vi "Array Outer Product (1D x 1D).vi"(1 "array a":dbl[](array[numeric])=[2.0, 1.0, 3.0], 4 "array b":dbl[](array[numeric])=[1.0, 2.0, 3.0]) -> (15 "a X b":dbl[][](array[numeric])=[[2.0, 4.0, 6.0], [1.0, 2.0, 3.0], [3.0, 6.0, 9.0]])   [LabVIEW 2014]
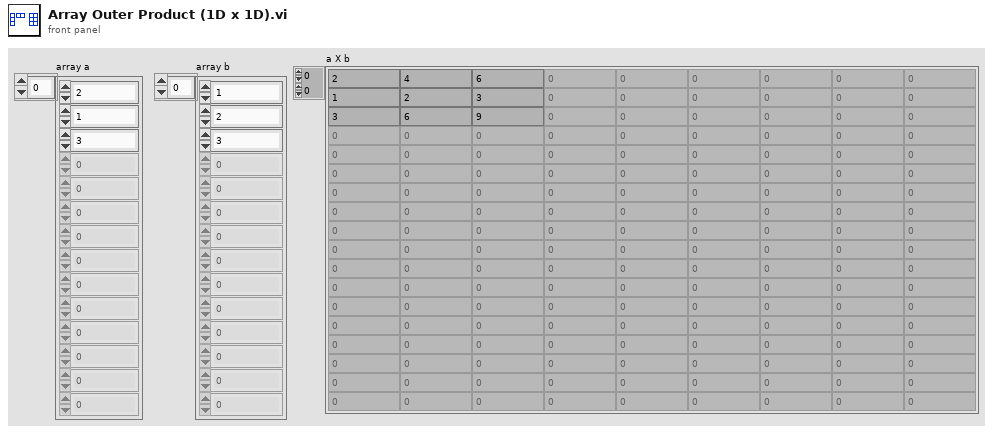
[diagram p1: front panel]
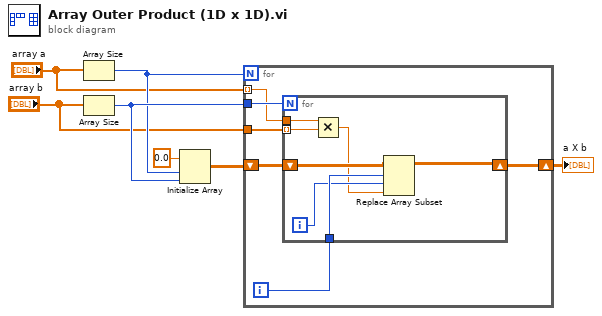
[diagram p0: block diagram]
diagram:
  n1 = Array Size(array="array a") -> (size(s)=w5:i32)
  n2 = Array Size(array="array b") -> (size(s)=w6:i32)
  n3 = Initialize Array(0.0 ("element"), w5, w6) -> (w2:dbl[][])
  n4 = for {
    N: w5 -> [_]
    shift-right: [w12] -> w7
    shift-left: w2 -> [w13]
    tunnel: "array a" -> [w9] mode=indexing
    tunnel: "array b" -> [w11]
    tunnel: w6 -> [w10]
    i -> [w8]
    n5 = for {
      N: w10 -> [_]
      shift-right: [w14] -> w12
      shift-left: w13 -> [w18]
      tunnel: w11 -> [w19] mode=indexing
      tunnel: w9 -> [w20]
      tunnel: w8 -> [w17]
      i -> [w16]
      n6 = Multiply(x=w20, y=w19) -> (x*y=w15:dbl)
      n7 = Replace Array Subset(array=w18, new element=w15, index (row)=w17, index (col)=w16) -> (w14:dbl[][])
    }
  }
  "a X b" <- w7
